vi "Update Methods Registration.vi"(8 "error in (no error)":errorcluster, 11 "Server class in":refnum<vi>) -> (0 "error out":errorcluster, 3 "Server class out":refnum<vi>)   [LabVIEW 2019, in "gRPC Scripting Tools.lvlib"]
uses:
  gRPC Scripting Tools.lvlib
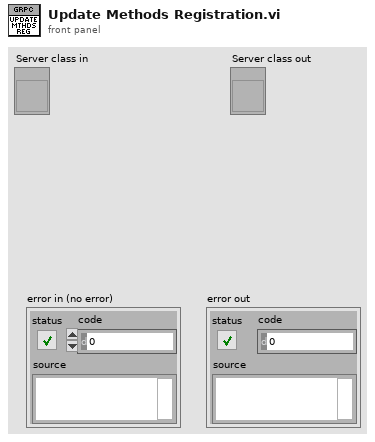
[diagram p1: front panel]
types:
  T1 = typedef "LVPointTypeDef.ctl" = cluster{"Horizontal":i16, "Vertical":i16}
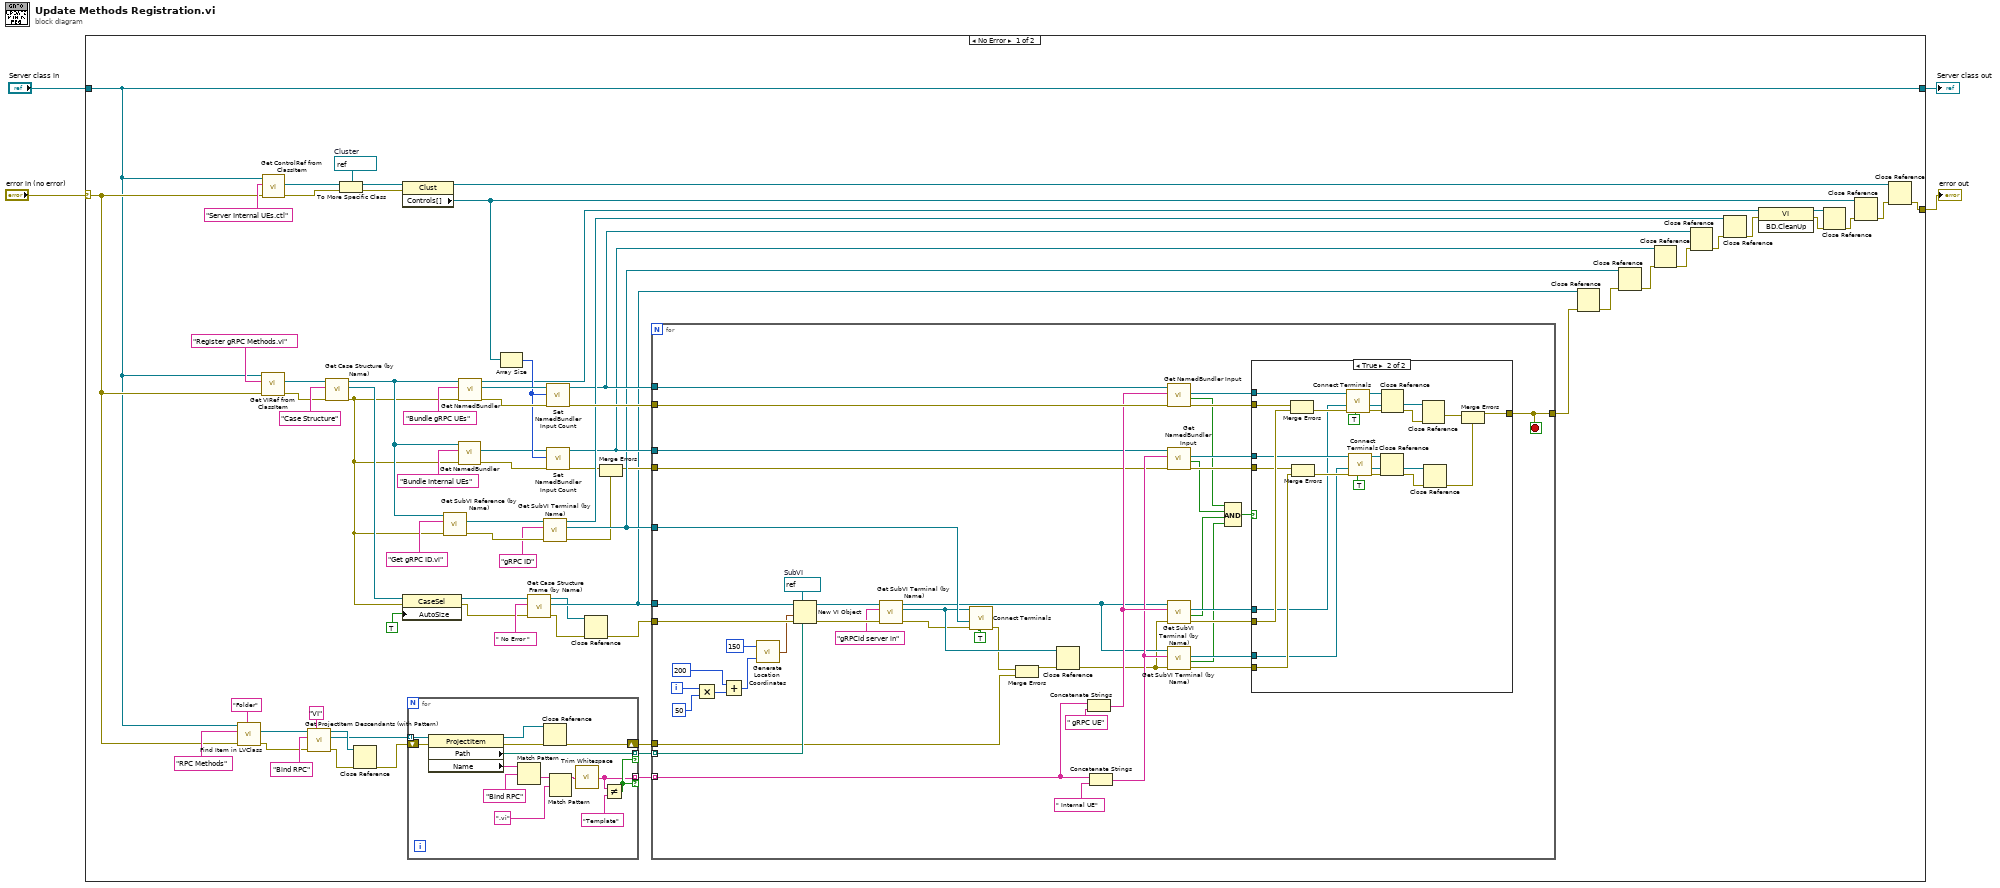
[diagram p0: block diagram]
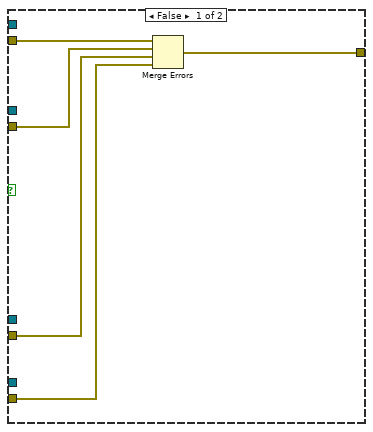
[diagram p2: hidden frame]
diagram:
  n1 = case shown="No Error" "error in (no error)" {
    selector: "error in (no error)" -> [w28 w158]
    tunnel: [w14 w158] -> w4
    tunnel: "Server class in" -> [w27 w159]
    tunnel: [w27 w159] -> w1
    frame No Error {
      w65 = refnum<vi> refnum  # Cluster
      n2 = call "Find Item in LVClass.vi"("Item Type"="Folder", "error in (no error)"=w28, "Item Name"="RPC Methods", "Class Item in"=w27) -> ("error out"=w39:errorcluster, "Project Item (Class Item)"=w40:refnum<vi>)  [unwired: 4 in, 2 out]
      n3 = call "Get VIRef from ClassItem.vi"("error in (no error)"=w28, "Item Name"="Register gRPC Methods.vi", "LVClassLibrary in"=w27) -> ("error out"=w59:errorcluster, "VIref out"=w72:refnum<vi>)  [unwired: 5 in, 2 out]
      n4 = call "Get ControlRef from ClassItem.vi"("error in (no error)"=w28, "Item Name"="Server Internal UEs.ctl", "LVClassLibrary in"=w27) -> ("error out"=w66:errorcluster, "Control ref out"=w64:refnum<vi>)  [unwired: 5 in, 2 out]
      n5 = call "Get ProjectItem Descendants (with Pattern).vi"("Type"="VI", "error in (no error)"=w39, "Pattern"="Bind RPC" ("regular expression"), "ProjectItem in"=w40) -> ("error out"=w38:errorcluster, "ProjectItem descendents"=w13:refnum<vi>[], "ProjectItem out"=w36:refnum<vi>)  [unwired: 5 in]
      n6 = call "Get Case Structure (by Name).vi"("error in (no error)"=w59, "Case Structure name"="Case Structure" ("y"), "VI ref in"=w72) -> ("error out"=w17:errorcluster, "CaseStructure out"=w21:refnum<vi>, "VI ref out"=w49:refnum<vi>)  [unwired: 5 in, 1 out]
      n7 = To More Specific Class(target class=w65, reference=w64, error in=w66) -> (specific class reference=w67:refnum<vi>, error out=w69:errorcluster)
      n8 = Close Reference(reference=w36, error in (no error)=w38) -> (error out=w10:errorcluster)
      n9 = property class="Clust"(reference=w67, error in=w69) -> (reference out=w16:refnum<vi>, "Controls[]"=w68:refnum<vi>[])  [unwired: 1 out]
      n10 = property class="CaseSel"(reference=w21, error in=w17, "AutoSize"=TRUE ("AutoSize To Fit Contents?")) -> (reference out=w20:refnum<vi>, error out=w19:errorcluster)
      n11 = for {
        tunnel: w13 -> [w87] mode=indexing
        tunnel: [w74] -> w11 mode=indexing if=w80
        tunnel: [w81] -> w12 mode=indexing if=w80
        shift-right: [w76] -> w9
        shift-left: w10 -> [w77]
        n12 = property class="ProjectItem"(reference=w87, error in=w77) -> (reference out=w78:refnum<vi>, error out=w79:errorcluster, "Path"=w81:path, "Name"=w83:string)
        n13 = Match Pattern(string=w83, regular expression="Bind RPC") -> (after substring=w85:string)  [unwired: 1 in, 3 out]
        n14 = Close Reference(reference=w78, error in (no error)=w79) -> (error out=w76:errorcluster)
        n15 = Match Pattern(string=w85, regular expression=".vi") -> (before substring=w75:string)  [unwired: 1 in, 3 out]
        n16 = call <vilib>:"Trim Whitespace.vi"("string"=w75) -> ("trimmed string"=w74:string)  [unwired: 1 in]
        n17 = Not Equal?(x=w74, y="Template") -> (x != y?=w80:bool)
      }
      n18 = call "Get SubVI Reference (by Name).vi"("error in (no error)"=w17, "SubVI Name"="Get gRPC ID.vi", "Owner VI in"=w49) -> ("error out"=w46:errorcluster, "SubVI Refnum out"=w47:refnum<vi>)  [unwired: 5 in, 2 out]
      n19 = call "Get NamedBundler.vi"("error in (no error)"=w17, "Label"="Bundle Internal UEs" ("name/order"), "Owner VI in"=w49) -> ("error out"=w50:errorcluster, "NamedBundler ref out"=w51:refnum<vi>)  [unwired: 5 in, 2 out]
      n20 = call "Get NamedBundler.vi"("error in (no error)"=w17, "Label"="Bundle gRPC UEs" ("name/order"), "Owner VI in"=w49) -> ("error out"=w53:errorcluster, "NamedBundler ref out"=w71:refnum<vi>, "Owner VI out"=w8:refnum<vi>)  [unwired: 5 in, 1 out]
      n21 = Array Size(array=w68) -> (size(s)=w52:i32)
      n22 = call "Get Case Structure Frame (by Name).vi"("error in (no error)"=w19, "element"=" No Error ", "CaseStructure in"=w20) -> ("error out"=w37:errorcluster, "Frame ref out"=w23:refnum<vi>, "CaseStructure out"=w22:refnum<vi>)  [unwired: 5 in, 1 out]
      n23 = call "Get SubVI Terminal (by Name).vi"("error in (no error)"=w46, "Terminal name"="gRPC ID", "SubVI in"=w47) -> ("error out"=w25:errorcluster, "SubVI Term ref"=w35:refnum<vi>, "SubVI out"=w44:refnum<vi>)  [unwired: 5 in, 1 out]
      n24 = call "Set NamedBundler Input Count.vi"("error in (no error)"=w53, "Numeric"=w52, "NamedBundler in"=w71) -> ("error out"=w61:errorcluster, "NamedBundler out"=w42:refnum<vi>)  [unwired: 7 in]
      n25 = call "Set NamedBundler Input Count.vi"("error in (no error)"=w50, "Numeric"=w52, "NamedBundler in"=w51) -> ("error out"=w26:errorcluster, "NamedBundler out"=w41:refnum<vi>)  [unwired: 7 in]
      n26 = Close Reference(reference=w22, error in (no error)=w37) -> (error out=w43:errorcluster)
      n27 = Merge Errors(w26, w25) -> (w24:errorcluster)
      n28 = for {
        tunnel: w23 -> [w133]
        tunnel: w61 -> [w132]
        tunnel: w42 -> [w131]
        tunnel: w43 -> [w125]
        tunnel: w24 -> [w121]
        tunnel: w41 -> [w122]
        tunnel: [w114] -> w34
        tunnel: w35 -> [w105]
        tunnel: w12 -> [w90] mode=indexing
        tunnel: w11 -> [w88] mode=indexing
        tunnel: w9 -> [w89]
        i -> [w102]
        stop <- w114 stop-if-true
        w130 = refnum<vi> refnum  # SubVI
        n29 = Multiply(x=w102, y=50) -> (x*y=w100:i32)
        n30 = Add(x=i16 200 ("Horizontal"), y=w100) -> (x+y=w98:i32)
        n31 = call "Generate Location Coordinates.vi"("Vertical"=w98, "Horizontal"=i16 150) -> ("Location out"=w97:T1)
        n32 = New VI Object(vi object class=w130, owner refnum=w133, position/next to=w97, 6:w90, 8:w125) -> (object refnum=w107:refnum<vi>, 0:w108:errorcluster)  [unwired: 3 in]
        n33 = call "Get SubVI Terminal (by Name).vi"("error in (no error)"=w108, "Terminal name"="gRPCid server in", "SubVI in"=w107) -> ("error out"=w94:errorcluster, "SubVI Term ref"=w95:refnum<vi>, "SubVI out"=w104:refnum<vi>)  [unwired: 5 in, 1 out]
        n34 = call "Connect Terminals.vi"("Auto Route? (F)"=TRUE, "Error In"=w94, "Source Terminal"=w105, "Sink Terminal"=w95) -> ("Error Out"=w92:errorcluster)  [unwired: 7 in]
        n35 = Merge Errors(w92, w89) -> (w91:errorcluster)
        n36 = Close Reference(reference=w95, error in (no error)=w91) -> (error out=w93:errorcluster)
        n37 = Concatenate Strings(w88, " gRPC UE" ("string")) -> (w126:string)
        n38 = Concatenate Strings(w88, " Internal UE" ("string")) -> (w123:string)
        n39 = call "Get NamedBundler Input.vi"("error in (no error)"=w132, "Input name"=w126, "NamedBundler ref in"=w131) -> ("error out"=w118:errorcluster, "Found?"=w113:bool, "Input Term ref"=w129:refnum<vi>)  [unwired: 5 in, 1 out]
        n40 = call "Get NamedBundler Input.vi"("error in (no error)"=w121, "Input name"=w123, "NamedBundler ref in"=w122) -> ("error out"=w116:errorcluster, "Found?"=w112:bool, "Input Term ref"=w120:refnum<vi>)  [unwired: 5 in, 1 out]
        n41 = call "Get SubVI Terminal (by Name).vi"("error in (no error)"=w93, "Terminal name"=w126, "SubVI in"=w104) -> ("error out"=w117:errorcluster, "Found?"=w111:bool, "SubVI Term ref"=w128:refnum<vi>)  [unwired: 5 in, 1 out]
        n42 = call "Get SubVI Terminal (by Name).vi"("error in (no error)"=w93, "Terminal name"=w123, "SubVI in"=w104) -> ("error out"=w115:errorcluster, "Found?"=w110:bool, "SubVI Term ref"=w119:refnum<vi>)  [unwired: 5 in, 1 out]
        n43 = Compound Arithmetic op=AND(w113, w112, w111, w110) -> (w109:bool)
        n44 = case shown="True" w109 {
          tunnel: w129 -> [_ w145]
          tunnel: w128 -> [_ w143]
          tunnel: w120 -> [_ w147]
          tunnel: w119 -> [_ w142]
          tunnel: w118 -> [w138 w157]
          tunnel: w117 -> [w135 w156]
          tunnel: w116 -> [w136 w155]
          tunnel: w115 -> [w134 w154]
          tunnel: [w137 w151] -> w114
          frame False {
            n45 = Merge Errors(w138, w136, w135, w134) -> (w137:errorcluster)
          }
          frame True {
            n46 = Merge Errors(w157, w156) -> (w153:errorcluster)
            n47 = Merge Errors(w155, w154) -> (w152:errorcluster)
            n48 = call "Connect Terminals.vi"("Auto Route? (F)"=TRUE, "Error In"=w153, "Source Terminal"=w143, "Sink Terminal"=w145) -> ("Error Out"=w146:errorcluster)  [unwired: 7 in]
            n49 = call "Connect Terminals.vi"("Auto Route? (F)"=TRUE, "Error In"=w152, "Source Terminal"=w142, "Sink Terminal"=w147) -> ("Error Out"=w148:errorcluster)  [unwired: 7 in]
            n50 = Close Reference(reference=w147, error in (no error)=w148) -> (error out=w141:errorcluster)
            n51 = Close Reference(reference=w145, error in (no error)=w146) -> (error out=w144:errorcluster)
            n52 = Close Reference(reference=w143, error in (no error)=w144) -> (error out=w140:errorcluster)
            n53 = Close Reference(reference=w142, error in (no error)=w141) -> (error out=w139:errorcluster)
            n54 = Merge Errors(w140, w139) -> (w151:errorcluster)
          }
        }
      }
      n55 = Close Reference(reference=w23, error in (no error)=w34) -> (error out=w33:errorcluster)
      n56 = Close Reference(reference=w35, error in (no error)=w33) -> (error out=w32:errorcluster)
      n57 = Close Reference(reference=w41, error in (no error)=w32) -> (error out=w31:errorcluster)
      n58 = Close Reference(reference=w42, error in (no error)=w31) -> (error out=w30:errorcluster)
      n59 = Close Reference(reference=w44, error in (no error)=w30) -> (error out=w7:errorcluster)
      n60 = invoke class="VI" method="BD.CleanUp"(reference=w8, error in=w7) -> (reference out=w6:refnum<vi>, error out=w5:errorcluster)  [unwired: 1 in, 1 out]
      n61 = Close Reference(reference=w6, error in (no error)=w5) -> (error out=w29:errorcluster)
      n62 = Close Reference(reference=w68, error in (no error)=w29) -> (error out=w15:errorcluster)
      n63 = Close Reference(reference=w16, error in (no error)=w15) -> (error out=w14:errorcluster)
    }
    frame Error {
    }
  }
  "error out" <- w4
  "Server class out" <- w1
